vi "FileOutput-Daemon.vi"(3 "Configuration":T1, 4 "OutputRequest\nuser event refnum":T2) -> ()   [LabVIEW 2015]
doc: "OutputRequest handler for the FileOutput output device. \n\nThis VI is meant to be started asynchronously. It will register itself as a listener on the OutputRequest user event refnum and process any requests that it knows how to handle.\n\nThe \"Configuration\" structure is used for initialization and contains:\n\"Logfile path\": Path to a logfile to create or append to\n\nCommands handled by this VI:\nTarget = \"all\"\n stop: Unregisters and stops running.\nTarget = \"\"timestamp\" or \"timestamped*\"\n [message];* Writes message to file along w/ system time"
uses:
  Typedefs/OutputRequest refnum.ctl
  Typedefs/OutputRequest.ctl
  FileOutput-Configuration.ctl
panel:
  out "File refnum":refnum<file>
  # "Just a local variable\nfor programming\nconvenience"
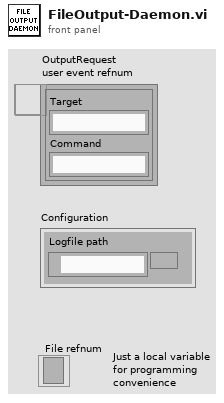
[diagram p1: front panel]
types:
  T1 = typedef "FileOutput-Configuration.ctl" = cluster{"Logfile path":path}
  T2 = typedef "OutputRequest refnum.ctl" = refnum<user-event>
  T3 = enum16{"open", "replace", "create", "open or create", "replace or create", "replace or create with confirmation"}
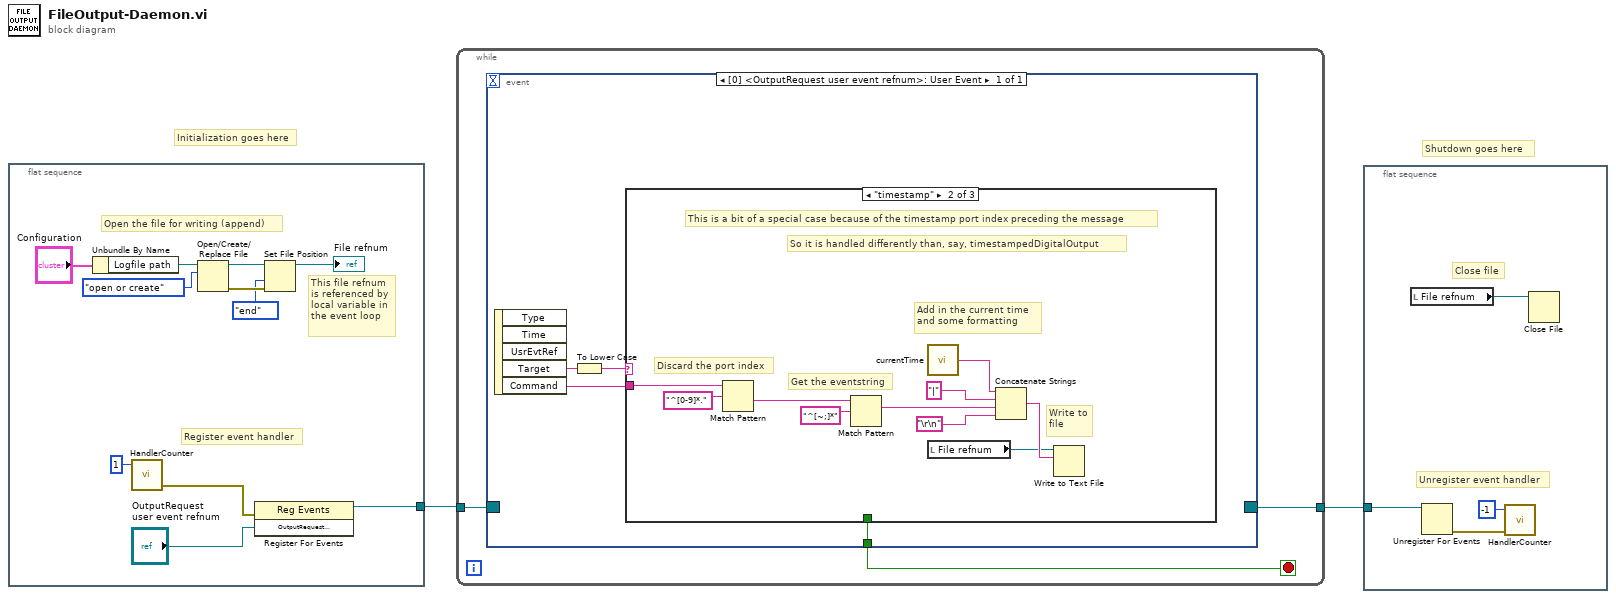
[diagram p0: block diagram]
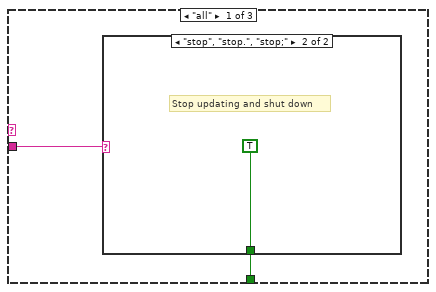
[diagram p2: hidden frame]
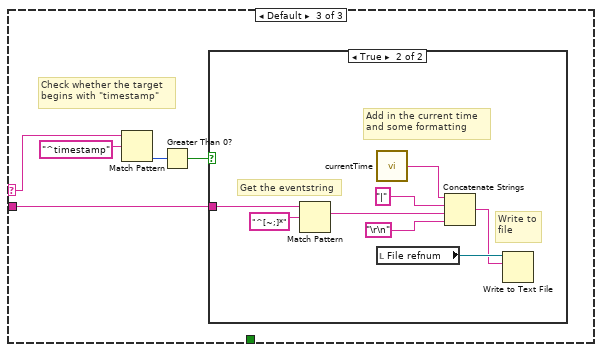
[diagram p4: hidden frame]
diagram:
  # "Shutdown goes here"
  # "Initialization goes here"
  n1 = flat-sequence {
    tunnel: [w13] -> w2
    frame #0 {
      # "Open the file for writing (append)"
      # "This file refnum\nis referenced by\nlocal variable in\nthe event loop"
      # "Register event handler"
      n2 = Unbundle By Name("Configuration") -> ("Logfile path"=w8:path)
      n3 = call "HandlerCounter.vi"("Change in count"=i16 1) -> ("error out"=w12:errorcluster)  [unwired: 3 in, 1 out]
      n4 = Open/Create/Replace File(file path (use dialog)=w8, operation (0:open)=T3."open or create") -> (refnum out=w7:refnum<file>, error out=w4:errorcluster)  [unwired: 4 in, 1 out]
      n5 = register-events(error in=w12, "OutputRequest\nuser event refnum") -> (reference out=w13:refnum<event-registration>)  [unwired: 1 in, 1 out]
      n6 = Set File Position(refnum=w7, from (0:start)=enum16{"start", "end", "current"}."end", error in=w4) -> (refnum out=→"File refnum":refnum<file>)  [unwired: 1 in, 1 out]
    }
  }
  n7 = while {
    tunnel: w2 -> [w16]
    tunnel: [w15] -> w1
    stop <- w14 stop-if-true
    n8 = event shown="[0] <OutputRequest\nuser event refnum>: User Event" {
      selector: w16 -> [_]
      dyn-events: [_] -> w15
      timeout: _ -> [_]
      tunnel: [w20] -> w14
      event User Event {
        n9 = event-data() -> ("Target"=w19:string, "Command"=w17:string)  [unwired: 1 in, 3 out]
        n10 = To Lower Case(string=w19) -> (all lower case string=w18:string)
        n11 = case shown="\"timestamp\"" w18 {
          selector: w18 -> [_ _ w37]
          tunnel: w17 -> [w22 w24 w34]
          tunnel: [w21 _ _] -> w20
          frame "all" {
            n12 = case shown="\"stop\", \"stop.\", \"stop;\"" w22 {
              tunnel: [_ TRUE] -> w21
              frame Default {
                # "We should probably put some\nerror throwing code here..."
              }
              frame "stop", "stop.", "stop;" {
                # "Stop updating and shut down"
              }
            }
          }
          frame "timestamp" {
            # "Discard the port index"
            # "Get the eventstring"
            # "Write to\nfile"
            # "Add in the current time\nand some formatting"
            # "So it is handled differently than, say, timestampedDigitalOutput"
            # "This is a bit of a special case because of the timestamp port index preceding the message"
            n13 = Match Pattern(string=w24, regular expression="^[0-9]*.") -> (after substring=w25:string)  [unwired: 1 in, 3 out]
            n14 = Match Pattern(string=w25, regular expression="^[~;]*") -> (match substring=w32:string)  [unwired: 1 in, 3 out]
            n15 = call "currentTime.vi"() -> ("String"=w27:string)
            n16 = local read "File refnum"() -> (w30:refnum<file>)
            n17 = Concatenate Strings(w27, "|" ("string"), w32, "\r\n") -> (w31:string)
            n18 = Write to Text File(file (use dialog)=w30, text=w31) -> ()  [unwired: 2 in, 3 out]
          }
          frame Default {
            # "Check whether the target\nbegins with \"timestamp\""
            n19 = Match Pattern(string=w37, regular expression="^timestamp") -> (offset past match=w36:i32)  [unwired: 1 in, 3 out]
            n20 = Greater Than 0?(x=w36) -> (x > 0?=w35:bool)
            n21 = case shown="True" w35 {
              tunnel: w34 -> [_ w40]
              frame False {
                # "Ignore the request, it doesn't pertain\nto this output device"
              }
              frame True {
                # "Get the eventstring"
                # "Write to\nfile"
                # "Add in the current time\nand some formatting"
                n22 = Match Pattern(string=w40, regular expression="^[~;]*") -> (match substring=w41:string)  [unwired: 1 in, 3 out]
                n23 = call "currentTime.vi"() -> ("String"=w46:string)
                n24 = local read "File refnum"() -> (w43:refnum<file>)
                n25 = Concatenate Strings(w46, "|" ("string"), w41, "\r\n") -> (w42:string)
                n26 = Write to Text File(file (use dialog)=w43, text=w42) -> ()  [unwired: 2 in, 3 out]
              }
            }
          }
        }
      }
    }
  }
  n27 = flat-sequence {
    tunnel: w1 -> [w50]
    frame #0 {
      # "Close file"
      # "Unregister event handler"
      n28 = local read "File refnum"() -> (w47:refnum<file>)
      n29 = Unregister For Events(event registration refnum=w50) -> (error out=w49:errorcluster)  [unwired: 1 in]
      n30 = call "HandlerCounter.vi"("error in"=w49, "Change in count"=i16 -1) -> ()  [unwired: 2 in, 2 out]
      n31 = Close File(refnum=w47) -> ()  [unwired: 1 in, 2 out]
    }
  }
